vi "Verify.vi"(8 "error in (no error)":errorcluster, 10 "Comparator":refnum<class "Comparator.lvclass">, 11 "Mock In":refnum<class "Responsive Mock.lvclass">) -> (0 "error out":errorcluster, 1 "Errors":errorcluster[](array[cluster]), 2 "Results":cluster{"Passed?":bool, "Message":string}[](array[cluster]))   [LabVIEW 2020, in "Responsive Mock.lvclass"]
uses:
  Responsive Mock.lvclass
  Comparator/Comparator.lvclass
  Responsive Mock.lvclass/Responsive Mock.ctl
  Expectation/Expectation.lvclass
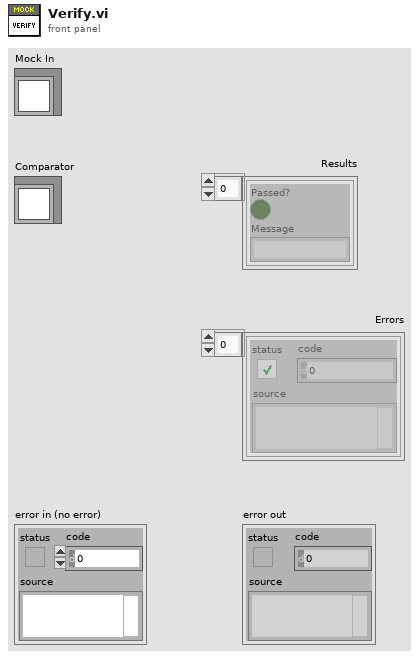
[diagram p1: front panel]
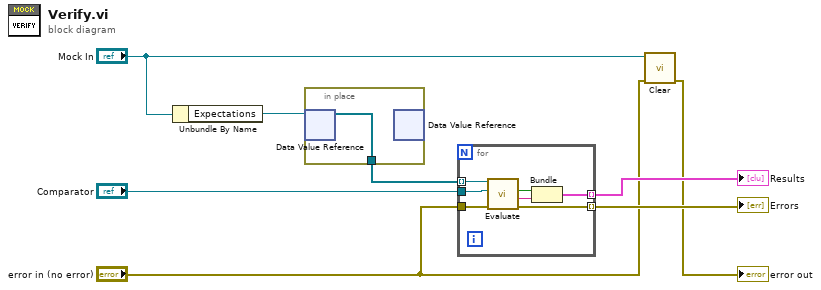
[diagram p0: block diagram]
diagram:
  n1 = Unbundle By Name("Mock In") -> ("Expectations"=w5:refnum<data-value>)
  n2 = in-place {
    in-place-border: [w9] -> w6
    n3 = in-place-dvr #1(w5) -> (w9:refnum<class "Expectation.lvclass">[])  [unwired: 1 out]
    n4 = in-place-dvr #1() -> ()  [unwired: 1 in, 2 out]
  }
  n5 = for {
    tunnel: "error in (no error)" -> [w16]
    tunnel: [w15] -> w8 mode=indexing
    tunnel: w6 -> [w14] mode=indexing
    tunnel: [w11] -> w7 mode=indexing
    tunnel: "Comparator" -> [w10]
    n6 = call-dynamic "Evaluate.vi"("error in (no error)"=w16, "Comparator"=w10, "Expectation in"=w14) -> ("error out"=w15:errorcluster, "Message"=w12:string, "Passed?"=w13:bool)  [unwired: 6 in]
    n7 = Bundle("Passed?"=w13, "Message"=w12) -> (w11:cluster{"Passed?":bool, "Message":string})  [unwired: 1 in]
  }
  "Errors" <- w8
  "Results" <- w7
  n8 = call-dynamic "Clear.vi"("error in (no error)"="error in (no error)", "Mock In"="Mock In") -> ("error out"=→"error out":errorcluster)  [unwired: 9 in]
